vi "Autonomous Independent.vi"() -> ()   [LabVIEW 2011]
doc: "This VI is called when autonomous begins, and will automatically be terminated when autonomous ends. You can carry out timed or sensor driven robot movement independently without needing to return to the caller."
uses:
  Robot Global Data.vi
  <vilib>/addons/control/pid/pid.llb/PID (DBL).vi
  <vilib>/Rock Robotics/WPI/Solenoid/Deprecated/WPI_SolenoidSetBool.vi
  <vilib>/addons/control/pid/NI_PID_pid.lvlib
panel:
  out "Auto State":T1(ring)
  out "Right":bool
  out "Center":bool
  out "Left":bool
  out "Mast encoder":dbl
  out "Drive train encoder":dbl
  out "gyro":dbl
  in  "Steering Gain":dbl=0.6
  # "Double line at end -- the T"
  # "This picture represents the robot following the left edge\nof the line.\nIt attempts to keep an edge sensor on the line,\nand all others off. This gives it three meaningful responses,\nsteer left, steer right, and go straight.\nThis allows for the other edge sensor to be used primarily\nfor identifying the T at the end of the line."
  # "Robot"
  # "Line"
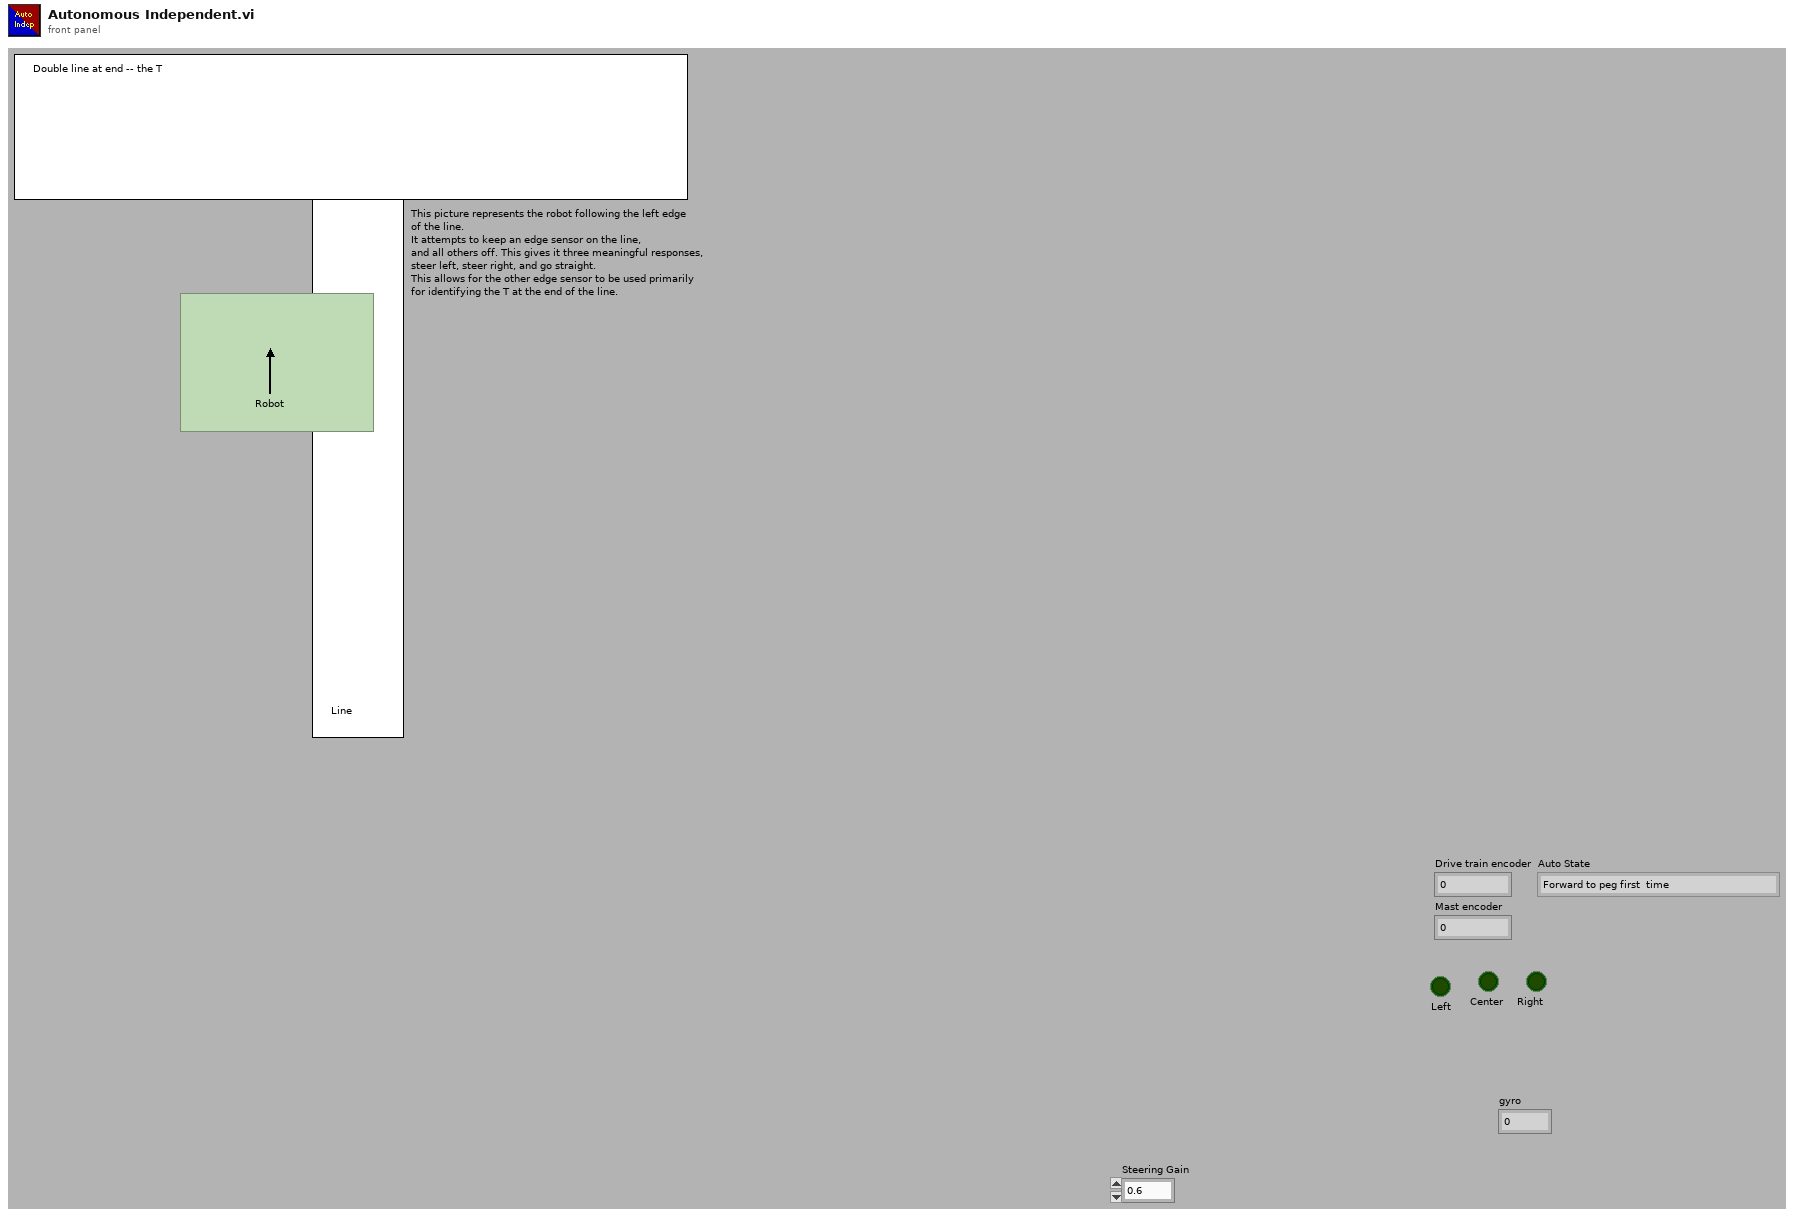
[diagram p1: front panel]
types:
  T1 = enum16{"Forward to peg first  time", "Lower Mast", "Open jaw", "Lower Mast again", "Back to second tube", "Spin to tube", "Forward to second tube", "Close jaw and forward", "Spin to zero gyro, face peg", "Forward to peg second time", "Lower mast 2", "Lower mast 3"}
  T2 = typedef "WPI_ServoDeviceRef.ctl" = cluster{"DeviceStatus":errorcluster, "Digital Module":T3, "PWM Channel":T4, "DeadBand":T5}
  T3 = typedef "FPGA_TypedefDigitalModule.ctl" = enum16{"Digital Module 1", "Digital Module 2"}
  T4 = typedef "FPGA_DIOPWMChannel.ctl" = enum8{"PWM 1", "PWM 2", "PWM 3", "PWM 4", "PWM 5", "PWM 6", "PWM 7", "PWM 8", "PWM 9", "PWM 10", "Invalid"}
  T5 = typedef "WPI_PWMDeadband.ctl" = cluster{"Name":string, "maxPositivePwm":i32, "minPositivePwm":i32, "centerPwm":i32, "maxNegativePwm":i32, "minNegativePwm":i32, "angularRange":u16}
  T6 = typedef "WPI_DigitalInputDevRef.ctl" = cluster{"DevStatus":errorcluster, "DIO Channel":T7, "Digital Module":T3}
  T7 = typedef "FPGA_DIOChannel.ctl" = enum8{"DIO 1", "DIO 2", "DIO 3", "DIO 4", "DIO 5", "DIO 6", "DIO 7", "DIO 8", "DIO 9", "DIO 10", "DIO 11", "DIO 12", "DIO 13", "DIO 14", "Invalid"}
  T8 = typedef "WPI_EncoderDevRef.ctl" = cluster{"DevStatus":errorcluster, "EncoderIndex":T9, "CounterIndex":T10, "DistancePerCount":dbl, "Decoding Type":T11}
  T9 = typedef "FPGA_EncoderIdx.ctl" = enum8{"Enc 0", "Enc 1", "Enc 2", "Enc 3", "Invalid"}
  T10 = typedef "FPGA_CounterCtrSystemIndex.ctl" = enum8{"Ctr 0", "Ctr 1", "Ctr 2", "Ctr 3", "Ctr 4", "Ctr 5", "Ctr 6", "Ctr 7", "Invalid"}
  T11 = typedef "WPI_EncoderType.ctl" = enum16{"1x", "2x", "4x"}
  T12 = typedef "WPI_RobotDriveDevRef.ctl" = cluster{"DevStatus":errorcluster, "Motors[]":T13[], "Square Inputs":bool, "Max Output":dbl}
  T13 = typedef "WPI_MotorControlDeviceRef.ctl" = cluster{"DeviceStatus":errorcluster, "Type":enum16{"PWM", "CAN"}, "PWM":cluster{"Digital Module":T3, "PWM Channel":T4, "DeadBand":T5}, "CAN":cluster{"Device Number":u8, "Control Mode":T14, "Semaphore":T15, "Max Vout":dbl}, "Invert":bool, "TransformRef":T16, "InvTransformRef":T16}
  T14 = typedef "WPI_CANJaguar_ControlMode.ctl" = enum8{"Percent VBus", "Current", "Speed", "Position", "Voltage"}
  T15 = typedef "Semaphore RefNum" = refnum<k1>
  T16 = typedef "WPI_PWMTransform_ConPane.ctl" = refnum<vi>
  T17 = typedef "WPI_GyroDevRef.ctl" = cluster{"DevStatus":errorcluster, "Analog Module":T18, "Analog Channel":T19, "Offset":dbl, "Gain (VoltsPerDegree/Second)":dbl}
  T18 = typedef "FPGA_TypedefAnalogModule.ctl" = enum16{"Analog Module 1", "Analog Module 2"}
  T19 = typedef "FPGA_AIChannel.ctl" = enum8{"AI 1", "AI 2", "AI 3", "AI 4", "AI 5", "AI 6", "AI 7", "AI 8", "Invalid"}
  T20 = typedef "WPI_SolenoidDevRef.ctl" = cluster{"DevStatus":errorcluster, "Solenoid Module":T21, "Forward Solenoid Channel":T22, "Reverse Solenoid Channel":T22}
  T21 = typedef "FPGA_TypedefSolenoidModule.ctl" = enum16{"Solenoid Module 1", "Solenoid Module 2"}
  T22 = typedef "WPI_SolenoidChannel.ctl" = enum8{"Solenoid 1", "Solenoid 2", "Solenoid 3", "Solenoid 4", "Solenoid 5", "Solenoid 6", "Solenoid 7", "Solenoid 8", "Invalid"}
  T23 = cluster{"Left":bool, "Center":bool, "Right":bool}
  T24 = cluster{"proportional gain (Kc)":dbl, "integral time (Ti, min)":dbl, "derivative time (Td, min)":dbl}
  T25 = enum16{"Forward to peg first  time", "Lower Mast", "Open jaw", "Lower Mast again", "Back to second tube", "Spin to tube", "Forward to second tube", "Close jaw and forward", "Spin to zero gyro, face peg", "Forward to peg second time", "Lower mast 2", "Lower mast 3", "Stop"}
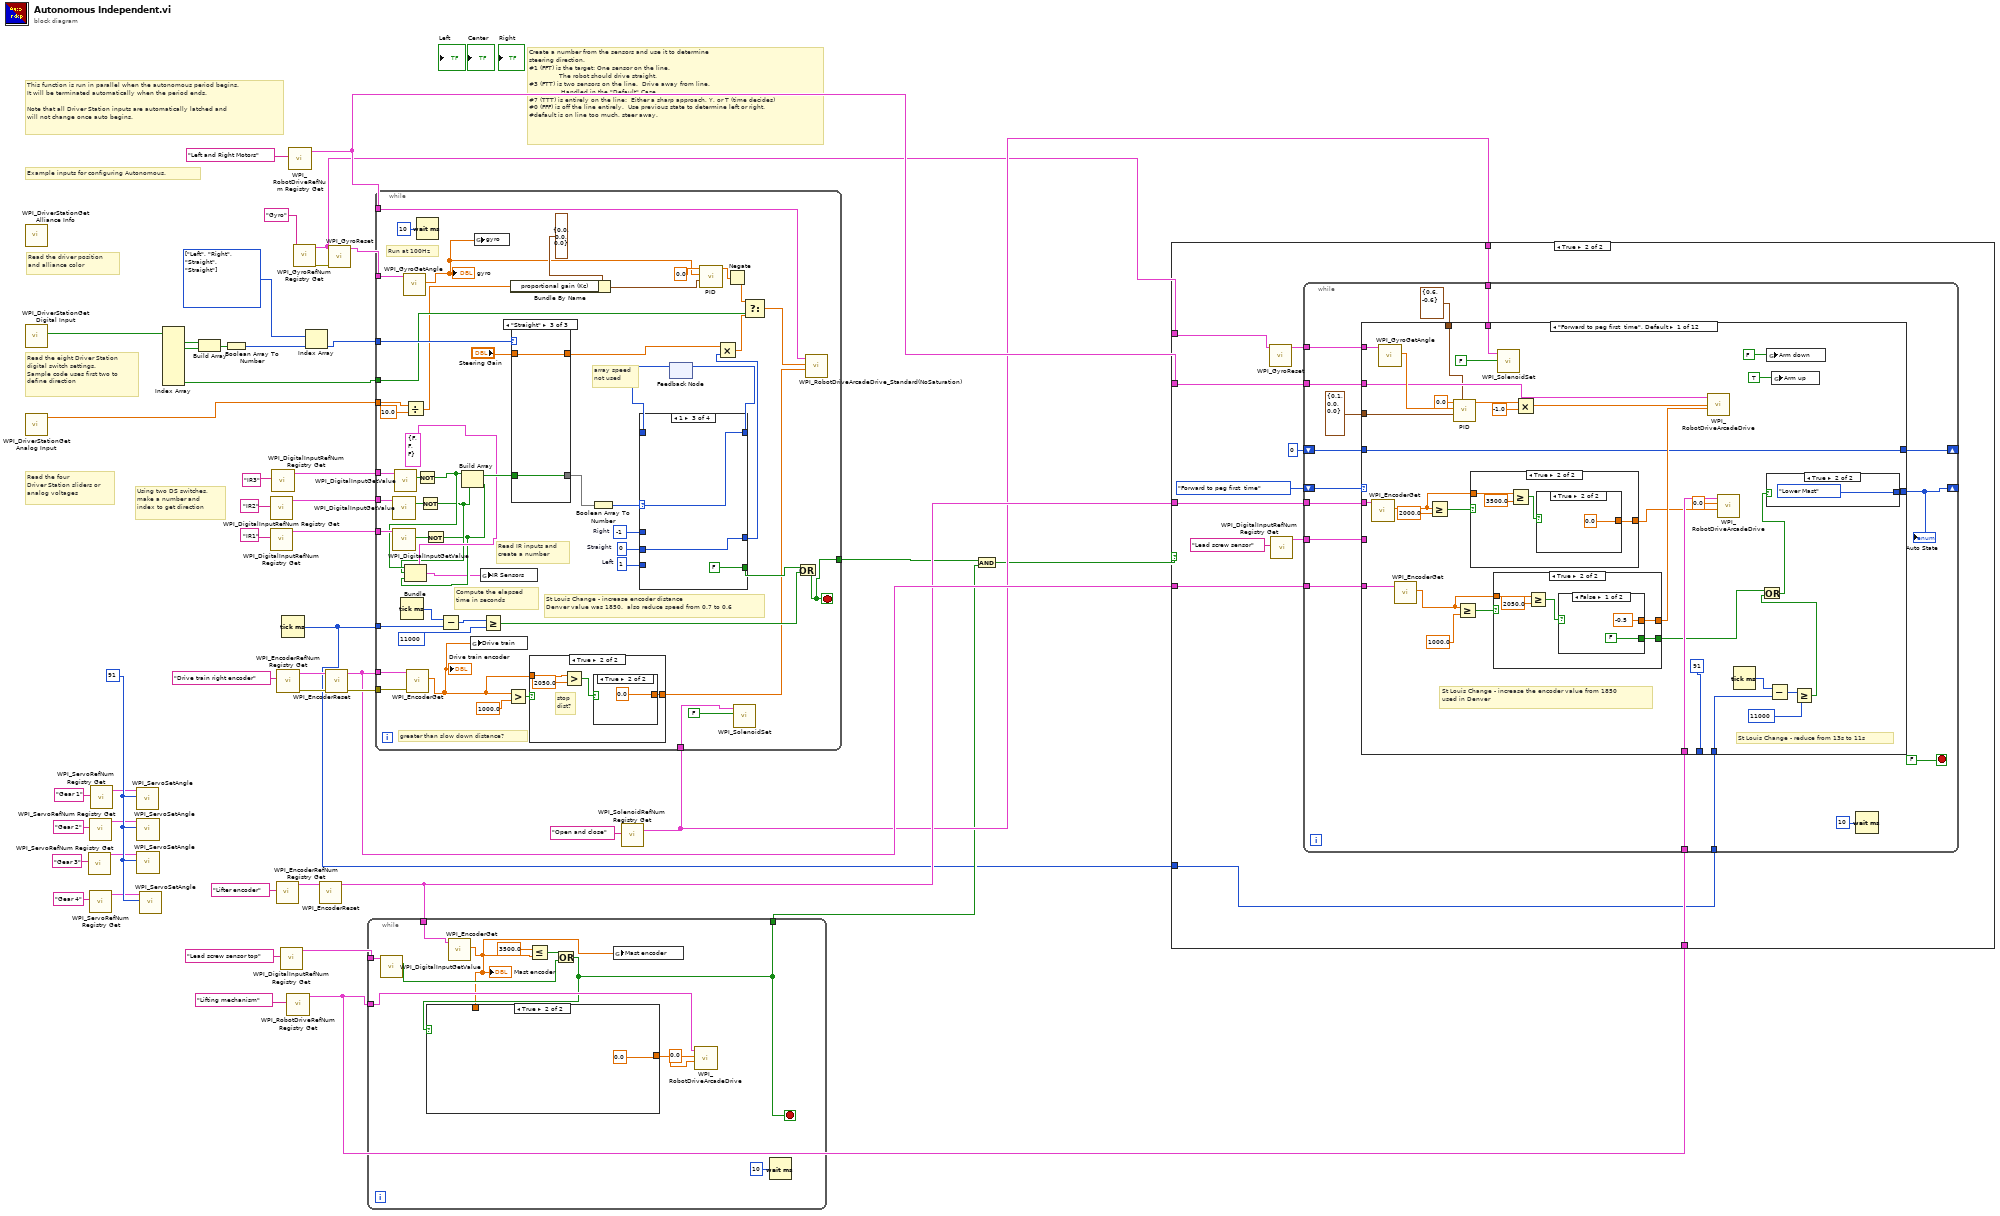
[diagram p0: block diagram]
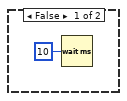
[diagram p2: hidden frame]
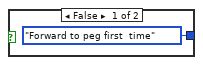
[diagram p3: hidden frame]
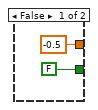
[diagram p4: hidden frame]
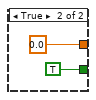
[diagram p5: hidden frame]
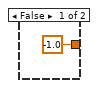
[diagram p6: hidden frame]
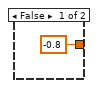
[diagram p7: hidden frame]
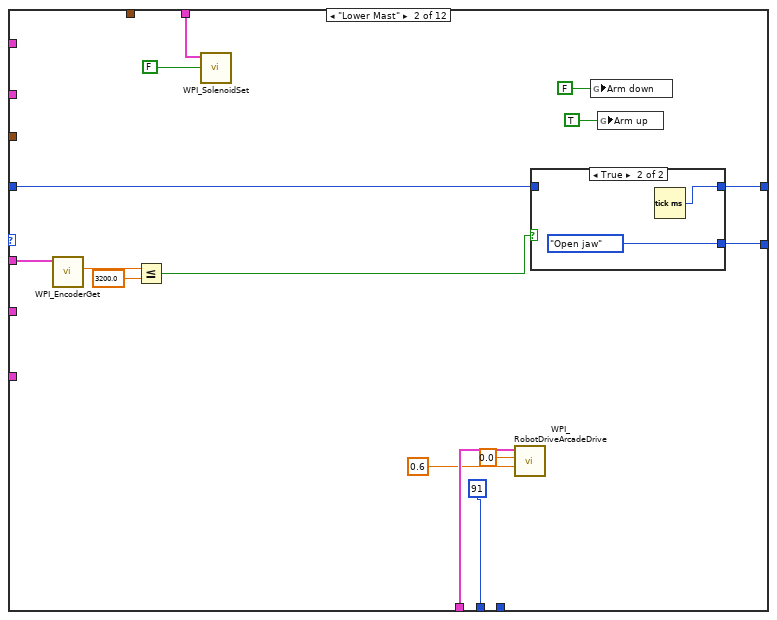
[diagram p8: hidden frame]
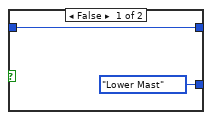
[diagram p9: hidden frame]
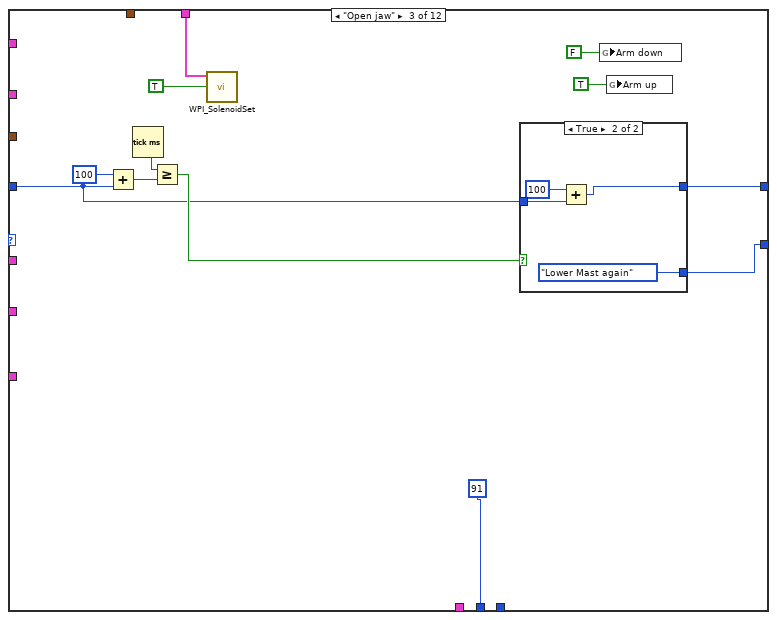
[diagram p10: hidden frame]
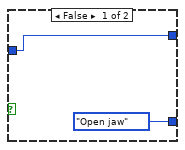
[diagram p11: hidden frame]
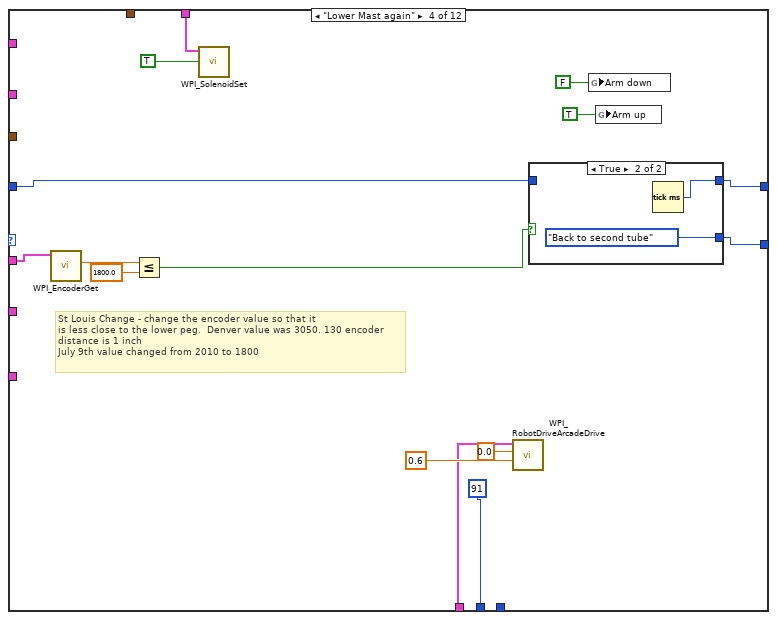
[diagram p12: hidden frame]
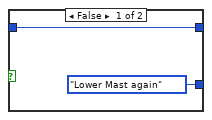
[diagram p13: hidden frame]
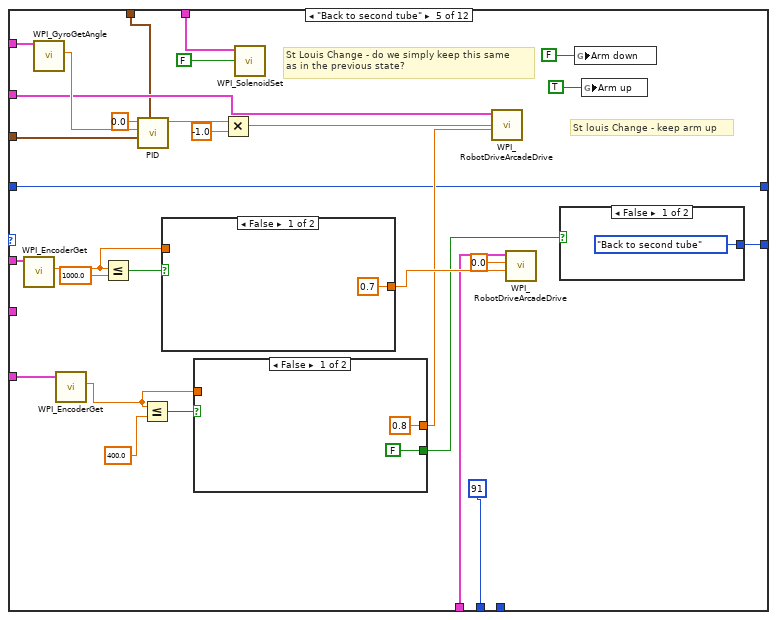
[diagram p14: hidden frame]
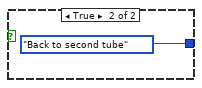
[diagram p15: hidden frame]
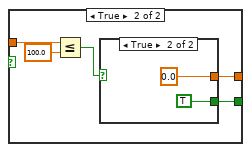
[diagram p16: hidden frame]
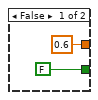
[diagram p17: hidden frame]
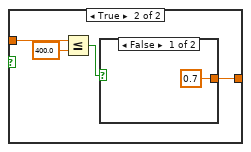
[diagram p18: hidden frame]
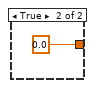
[diagram p19: hidden frame]
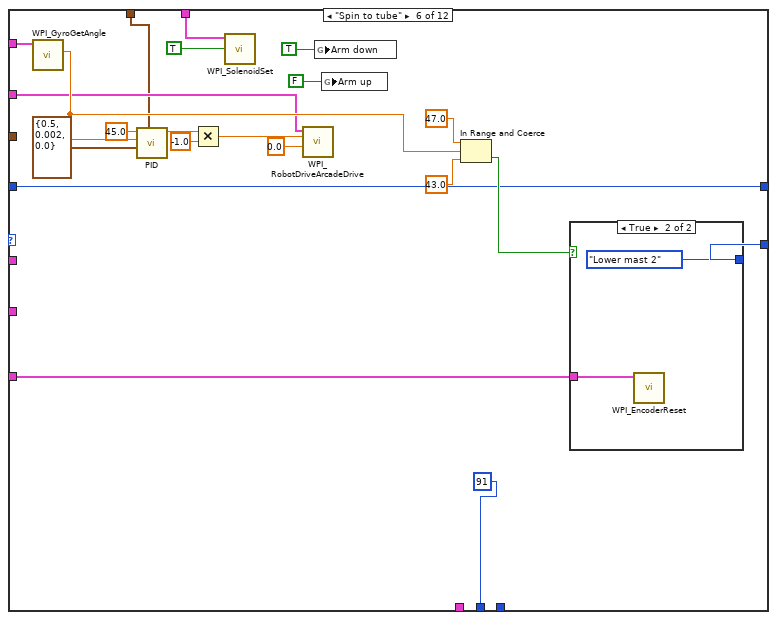
[diagram p20: hidden frame]
diagram:
  w24 = 91 ("Angle")
  w43 = enum16{"Left", "Right", "Straight"}[] [enum."Left", enum."Right", enum."Straight", enum."Straight"] items=["Left", "Right", "Straight"]
  # "Create a number from the sensors and use it to determine\nsteering direction.\n#1 (FFT) is the target: One sensor on the line.  \n               The robot should drive straight.\n#3 (FTT) is two sensors on the line.  Drive away from line.\n                Handled in the \"Default\" Case.\n#7 (TTT) is entirely on the line:  Either a sharp approach, Y, or T (time decides)\n#0 (FFF) is off the line entirely.  Use previous state to determine left or right. \n#default is on line too much, steer away."
  # "Using two DS switches,\nmake a number and\nindex to get direction"
  # "Example inputs for configuring Autonomous."
  # "Read the driver position\nand alliance color"
  # "Read the eight Driver Station\ndigital switch settings.\nSample code uses first two to\ndefine direction"
  # "Read the four\nDriver Station sliders or\nanalog voltages"
  # "This function is run in parallel when the autonomous period begins.\nIt will be terminated automatically when the period ends.\n\nNote that all Driver Station inputs are automatically latched and\nwill not change once auto begins."
  n1 = call <vilib>:"WPI_DriverStationGet Alliance Info.vi"() -> ()  [unwired: 12 out]
  n2 = call <vilib>:"WPI_DriverStationGet Digital Input.vi"() -> ("Driver Station Digital Input (1-8)"=w48:bool[])  [unwired: 11 out]
  n3 = call <vilib>:"WPI_DriverStationGet Analog Input.vi"() -> ("Analog 1 (V)"=w1:dbl)  [unwired: 11 out]
  n4 = call <vilib>:"WPI_ServoRefNum Registry Get.vi"("refnum name"="Gear 3") -> ("ServoDeviceRef"=w17:T2)  [unwired: 1 in, 9 out]
  n5 = call <vilib>:"WPI_ServoRefNum Registry Get.vi"("refnum name"="Gear 2") -> ("ServoDeviceRef"=w18:T2)  [unwired: 1 in, 9 out]
  n6 = call <vilib>:"WPI_ServoRefNum Registry Get.vi"("refnum name"="Gear 4") -> ("ServoDeviceRef"=w16:T2)  [unwired: 1 in, 9 out]
  n7 = call <vilib>:"WPI_ServoRefNum Registry Get.vi"("refnum name"="Gear 1") -> ("ServoDeviceRef"=w19:T2)  [unwired: 1 in, 9 out]
  n8 = call <vilib>:"WPI_ServoSetAngle.vi"("Angle"=w24, "ServoDeviceRef"=w19) -> ()  [unwired: 1 in, 9 out]
  n9 = call <vilib>:"WPI_ServoSetAngle.vi"("Angle"=w24, "ServoDeviceRef"=w18) -> ()  [unwired: 1 in, 9 out]
  n10 = call <vilib>:"WPI_ServoSetAngle.vi"("Angle"=w24, "ServoDeviceRef"=w17) -> ()  [unwired: 1 in, 9 out]
  n11 = call <vilib>:"WPI_ServoSetAngle.vi"("Angle"=w24, "ServoDeviceRef"=w16) -> ()  [unwired: 1 in, 9 out]
  n12 = Index Array(array=w48) -> (element #1=w46:bool, element #2=w45:bool, element #8=w4:bool)  [unwired: 8 in, 5 out]
  n13 = Build Array(w46, w45) -> (w44:bool[])
  n14 = Boolean Array To Number(Boolean array=w44) -> (number=w42:u32)
  n15 = call <vilib>:"WPI_DigitalInputRefNum Registry Get.vi"("refnum name"="IR2") -> ("DigitalInputDevRef"=w29:T6)  [unwired: 1 in, 9 out]
  n16 = call <vilib>:"WPI_DigitalInputRefNum Registry Get.vi"("refnum name"="IR1") -> ("DigitalInputDevRef"=w28:T6)  [unwired: 1 in, 9 out]
  n17 = call <vilib>:"WPI_DigitalInputRefNum Registry Get.vi"("refnum name"="IR3") -> ("DigitalInputDevRef"=w30:T6)  [unwired: 1 in, 9 out]
  n18 = call <vilib>:"WPI_EncoderRefNum Registry Get.vi"("refnum name"="Lifter encoder") -> ("EncoderDevRef"=w25:T8)  [unwired: 1 in, 9 out]
  n19 = call <vilib>:"WPI_EncoderRefNum Registry Get.vi"("refnum name"="Drive train right encoder") -> ("error out"=w32:errorcluster, "EncoderDevRef"=w31:T8)  [unwired: 1 in, 8 out]
  n20 = call <vilib>:"WPI_DigitalInputRefNum Registry Get.vi"("refnum name"="Lead screw sensor top") -> ("DigitalInputDevRef"=w26:T6)  [unwired: 1 in, 9 out]
  n21 = Tick Count (ms)() -> (millisecond timer value=w8:u32)
  n22 = call <vilib>:"WPI_RobotDriveRefNum Registry Get.vi"("refnum name"="Lifting mechanism") -> ("RobotDriveDevRef"=w14:T12)  [unwired: 1 in, 9 out]
  n23 = call <vilib>:"WPI_RobotDriveRefNum Registry Get.vi"("refnum name"="Left and Right Motors") -> ("RobotDriveDevRef"=w15:T12)  [unwired: 1 in, 9 out]
  n24 = call <vilib>:"WPI_GyroRefNum Registry Get.vi"("refnum name"="Gyro") -> ("error out"=w7:errorcluster, "GyroDevRef"=w3:T17)  [unwired: 1 in, 8 out]
  n25 = Index Array(array=w43, index=w42) -> (element=w37:enum16{"Left", "Right", "Straight"})
  n26 = call <vilib>:"WPI_EncoderReset.vi"("EncoderDevRef"=w25) -> ("EncoderDevRef"=w12:T8)  [unwired: 1 in, 9 out]
  n27 = call <vilib>:"WPI_EncoderReset.vi"("error in (no error)"=w32, "EncoderDevRef"=w31) -> ("error out"=w27:errorcluster, "EncoderDevRef"=w13:T8)  [unwired: 8 out]
  n28 = call <vilib>:"WPI_GyroReset.vi"("error in (no error)"=w7, "GyroDevRef"=w3) -> ("GyroDevRef"=w5:T17)  [unwired: 9 out]
  n29 = while {
    tunnel: w14 -> [w57]
    tunnel: w26 -> [w59]
    tunnel: [w51] -> w10
    tunnel: w12 -> [w56]
    stop <- w51 stop-if-true
    n30 = call <vilib>:"WPI_DigitalInputGetValue.vi"("DigitalInputDevRef"=w59) -> ("Value"=w52:bool)  [unwired: 1 in, 9 out]
    n31 = call <vilib>:"WPI_EncoderGet.vi"("EncoderDevRef"=w56) -> ("Distance"=w50:dbl)  [unwired: 1 in, 9 out]
    "Mast encoder" <- w50
    n32 = Less Or Equal?(x=3500.0, y=w50) -> (x <= y?=w53:bool)
    n33 = Or(x=w53, y=w52) -> (x .or. y?=w51:bool)
    n34 = case shown="True" w51 {
      tunnel: [w63 0.0 ("Y axis value")] -> w55
      tunnel: w50 -> [w60 _]
      frame False {
        # "slow down if encoder is 2700"
        n35 = Greater Or Equal?(x=w60, y=2700.0) -> (x >= y?=w62:bool)
        n36 = case shown="True" w62 {
          tunnel: [-1.0 ("Y axis value") -0.6 ("Y axis value")] -> w63
          frame False {
          }
          frame True {
          }
        }
      }
      frame True {
      }
    }
    n37 = global write "Robot Global Data.vi" "Mast encoder"(w50) -> ()
    n38 = call-poly <vilib>:"WPI_RobotDriveArcadeDrive.vi"("Y axis value"=w55, "X axis value"=0.0, "RobotDriveDevRef"=w57) -> ()  [unwired: 1 in, 8 out]
    n39 = Wait (ms)(milliseconds to wait=u32 10) -> ()  [unwired: 1 out]
  }
  n40 = call <vilib>:"WPI_SolenoidRefNum Registry Get.vi"("refnum name"="Open and close") -> ("SolenoidDevRef"=w11:T20)  [unwired: 1 in, 9 out]
  n41 = while {
    tunnel: w15 -> [w99]
    tunnel: w30 -> [w119]
    tunnel: w29 -> [w118]
    tunnel: w28 -> [w117]
    tunnel: w8 -> [w78]
    tunnel: w37 -> [w103]
    tunnel: w13 -> [w98]
    tunnel: w27 -> [w97]
    tunnel: w11 -> [w93]
    tunnel: w5 -> [w92]
    tunnel: w4 -> [w86]
    tunnel: [w75] -> w2
    tunnel: w1 -> [w72]
    stop <- w75 stop-if-true
    w111 = 0  # Straight
    w110 = 1  # Left
    w112 = -1  # Right
    # "St Louis Change - increase encoder distance \nDenver value was 1850.  also reduce speed from 0.7 to 0.6"
    # "array speed\nnot used"
    # "greater than slow down distance?"
    # "Run at 100Hz"
    # "Read IR inputs and\ncreate a number"
    # "Compute the elapsed\ntime in seconds"
    n42 = call <vilib>:"WPI_DigitalInputGetValue.vi"("DigitalInputDevRef"=w118) -> ("Value"=w101:bool)  [unwired: 1 in, 9 out]
    n43 = call <vilib>:"WPI_DigitalInputGetValue.vi"("DigitalInputDevRef"=w117) -> ("Value"=w100:bool)  [unwired: 1 in, 9 out]
    n44 = call <vilib>:"WPI_DigitalInputGetValue.vi"("DigitalInputDevRef"=w119) -> ("Value"=w102:bool)  [unwired: 1 in, 9 out]
    n45 = Tick Count (ms)() -> (millisecond timer value=w109:u32)
    n46 = call <vilib>:"WPI_GyroGetAngle.vi"("GyroDevRef"=w92) -> ("Angle"=w85:dbl)  [unwired: 1 in, 9 out]
    "gyro" <- w85
    n47 = Divide(x=w72, y=10.0) -> (x/y=w71:dbl)
    n48 = call <vilib>:"WPI_EncoderGet.vi"("error in (no error)"=w97, "EncoderDevRef"=w98) -> ("Distance"=w69:dbl)  [unwired: 9 out]
    "Drive train encoder" <- w69
    n49 = Not(x=w102) -> (.not. x?=w83:bool)
    n50 = Wait (ms)(milliseconds to wait=u32 10) -> ()  [unwired: 1 out]
    n51 = Not(x=w101) -> (.not. x?=w82:bool)
    n52 = Not(x=w100) -> (.not. x?=w81:bool)
    n53 = Bundle(cluster=T23 {"Left"=FALSE, "Center"=FALSE, "Right"=FALSE} ("IR Sensors"), "Left"=w83, "Center"=w82, "Right"=w81) -> (w80:T23)
    n54 = Subtract(x=w109, y=w78) -> (x-y=w77:u32)
    n55 = Build Array(w83, w82, w81) -> (w108:bool[])
    n56 = global write "Robot Global Data.vi" "Drive train"(w69) -> ()
    n57 = global write "Robot Global Data.vi" "gyro"(w85) -> ()
    n58 = global write "Robot Global Data.vi" "IR Sensors"(w80) -> ()
    n59 = Greater Or Equal?(x=w77, y=u32 11000 ("milliseconds to wait")) -> (x >= y?=w76:bool)
    n60 = Greater?(x=w69, y=1000.0) -> (0:w95:bool)
    n61 = Bundle By Name(cluster=T24 {"proportional gain (Kc)"=0.0, "integral time (Ti, min)"=0.0, "derivative time (Td, min)"=0.0} ("PID gains"), "proportional gain (Kc)"=w71) -> (w89:T24)
    n62 = case shown="\"Straight\"" w103 {
      tunnel: w108 -> [w127 w130 w133]
      tunnel: [w127 w129 w133] -> w107
      tunnel: "Steering Gain" -> [w128 w132 w134]
      tunnel: [w128 w131 w134] -> w104
      frame "Left", Default {
      }
      frame "Right" {
        n63 = Negate(x=w132) -> (-x=w131:dbl)
        n64 = Reverse 1D Array(array=w130) -> (reversed array=w129:bool[])
      }
      frame "Straight" {
      }
    }
    n65 = case shown="True" w95 {
      tunnel: [-0.7 ("Y axis value") w123] -> w74
      tunnel: w69 -> [_ w121]
      frame False {
      }
      frame True {
        # "stop\ndist?"
        n66 = Greater?(x=w121, y=2050.0) -> (0:w122:bool)
        n67 = case shown="True" w122 {
          tunnel: [-0.5 ("Y axis value") 0.0 ("Y axis value")] -> w123
          frame False {
          }
          frame True {
          }
        }
      }
    }
    n68 = Boolean Array To Number(Boolean array=w107) -> (number=w116:u32)
    n69 = feedback #1() -> (w115:u32)  [unwired: 1 out]
    n70 = case shown="1" w116 {
      selector: w116 -> [w136 _ w147 w150]
      tunnel: w112 -> [_ w140 _ _]
      tunnel: w111 -> [_ _ w148 w151]
      tunnel: w110 -> [w137 w141 _ _]
      tunnel: [w137 w139 w148 w151] -> w106
      tunnel: w115 -> [_ w142 _ _]
      tunnel: [w136 w142 w147 w150] -> w114
      tunnel: [FALSE FALSE FALSE TRUE] -> w79
      frame Default {
      }
      frame 0 {
        # "#1-exited on right\n#7-inside Y\n#0 initial condition"
        n71 = case shown="0, 1" w142 {
          tunnel: w141 -> [w143 _ w145]
          tunnel: w140 -> [_ w144 _]
          tunnel: [w143 w144 w145] -> w139
          frame Default {
          }
          frame 0, 1 {
          }
          frame 7 {
          }
        }
      }
      frame 1 {
      }
      frame 7 {
      }
    }
    n72 = feedback-in #1(w114) -> ()
    n73 = call-poly <vilib>:"PID.vi"("PID gains"=w89, "process variable"=w85, "setpoint"=0.0) -> ("output"=w68:dbl)  [unwired: 3 in, 5 out]
    n74 = Multiply(x=w104, y=w106) -> (x*y=w88:dbl)
    n75 = Negate(x=w68) -> (-x=w67:dbl)
    n76 = call-poly <vilib>:"WPI_SolenoidSet.vi"("Value"=FALSE, "SolenoidDevRef"=w93) -> ()  [unwired: 1 in, 9 out]
    n77 = Select(t=w67, s=w86, f=w88) -> (s? t:f=w87:dbl)
    n78 = Or(x=w79, y=w76) -> (x .or. y?=w75:bool)
    n79 = call <vilib>:"WPI_RobotDriveArcadeDrive_Standard(NoSaturation).vi"("Y axis value"=w74, "X axis value"=w87, "RobotDriveDevRef"=w99) -> ()  [unwired: 1 in, 8 out]
  }
  n80 = And(x=w2, y=w10) -> (x .and. y?=w9:bool)
  n81 = case shown="True" w9 {
    tunnel: w15 -> [_ w159]
    tunnel: w14 -> [_ w158]
    tunnel: w13 -> [_ w157]
    tunnel: w12 -> [_ w156]
    tunnel: w11 -> [_ w155]
    tunnel: w8 -> [_ w154]
    tunnel: w3 -> [_ w153]
    frame False {
      n82 = Wait (ms)(milliseconds to wait=u32 10) -> ()  [unwired: 1 out]
    }
    frame True {
      n83 = call <vilib>:"WPI_GyroReset.vi"("GyroDevRef"=w153) -> ("GyroDevRef"=w163:T17)  [unwired: 10 out]
      n84 = call <vilib>:"WPI_DigitalInputRefNum Registry Get.vi"("refnum name"="Lead screw sensor") -> ("DigitalInputDevRef"=w160:T6)  [unwired: 1 in, 9 out]
      n85 = while {
        shift-right: [w172] -> _
        shift-left: T25."Forward to peg first  time" -> [w179]
        tunnel: w163 -> [w178]
        tunnel: w159 -> [w176]
        tunnel: w157 -> [w175]
        tunnel: w156 -> [w174]
        tunnel: w158 -> [w173]
        shift-right: [w170] -> _
        shift-left: u32 0 ("millisecond timer value") -> [w171]
        tunnel: w155 -> [w169]
        tunnel: w160 -> [w168]
        tunnel: w154 -> [w166]
        stop <- FALSE stop-if-true
        n86 = case shown="\"Forward to peg first  time\", Default" w179 {
          tunnel: w178 -> [w215 _ _ _ w303 w356 w383 w411 w435 w462 _ _]
          tunnel: T24 {"proportional gain (Kc)"=0.1, "integral time (Ti, min)"=0.0, "derivative time (Td, min)"=0.0} ("PID gains") -> [w212 _ _ _ w302 _ w384 w410 _ w460 _ _]
          tunnel: w176 -> [w211 _ _ _ w304 w344 w382 w412 w434 w461 _ _]
          tunnel: w175 -> [w210 _ _ _ w299 w343 w377 w407 w430 w458 _ _]
          tunnel: w174 -> [w209 w250 _ w278 w295 _ _ _ _ w459 w505 w524]
          tunnel: w173 -> [w202 w245 _ w275 w300 _ w366 _ _ w456 w508 w521]
          tunnel: [w199 w246 w263 w277 w297 w347 w374 w403 w431 w455 w506 T1."Lower mast 3"] -> w172
          tunnel: w171 -> [w196 w239 w261 w279 w301 w345 w375 w405 w433 w457 w509 _]
          tunnel: [w196 w240 w260 w276 w301 w345 w375 w405 w433 w457 w507 u32 0 ("millisecond timer value")] -> w170
          tunnel: w169 -> [w194 w237 w259 w274 w296 w353 w385 w413 w436 w463 w501 w528]
          tunnel: w168 -> [_ _ _ _ _ _ w367 _ _ _ _ _]
          tunnel: cluster{"output high":dbl, "output low":dbl} {"output high"=0.6, "output low"=-0.6} ("output range") -> [w190 _ _ _ w294 w342 w372 w402 w429 w454 _ _]
          tunnel: [91 ("Angle") 91 ("Angle") 91 ("Angle") 91 ("Angle") 91 ("Angle") 91 ("Angle") 91 ("Angle") 91 ("Angle") 91 ("Angle") 91 ("Angle") 91 ("Angle") 91 ("Angle")] -> _
          tunnel: w166 -> [w186 _ _ _ _ _ _ _ _ _ _ _]
          frame "Forward to peg first  time", Default {
            # "St Louis Change - reduce from 13s to 11s"
            # "St Louis Change - increase the encoder value from 1850\nused in Denver"
            n87 = call <vilib>:"WPI_EncoderGet.vi"("EncoderDevRef"=w209) -> ("Distance"=w200:dbl)  [unwired: 1 in, 9 out]
            n88 = call <vilib>:"WPI_GyroGetAngle.vi"("GyroDevRef"=w215) -> ("Angle"=w214:dbl)  [unwired: 1 in, 9 out]
            n89 = call <vilib>:"WPI_EncoderGet.vi"("EncoderDevRef"=w210) -> ("Distance"=w188:dbl)  [unwired: 1 in, 9 out]
            n90 = Greater Or Equal?(x=w200, y=2000.0) -> (x >= y?=w207:bool)
            n91 = call-poly <vilib>:"PID.vi"("output range"=w190, "PID gains"=w212, "process variable"=w214, "setpoint"=0.0) -> ("output"=w193:dbl)  [unwired: 2 in, 5 out]
            n92 = Greater Or Equal?(x=w188, y=1000.0) -> (x >= y?=w206:bool)
            n93 = case shown="True" w207 {
              tunnel: [-1.0 ("Y axis value") w233] -> w201
              tunnel: w200 -> [_ w232]
              frame False {
              }
              frame True {
                n94 = Greater Or Equal?(x=w232, y=3500.0) -> (x >= y?=w230:bool)
                n95 = case shown="True" w230 {
                  tunnel: [-0.8 ("Y axis value") 0.0 ("Y axis value")] -> w233
                  frame False {
                  }
                  frame True {
                  }
                }
              }
            }
            n96 = case shown="True" w206 {
              tunnel: [-0.5 ("Y axis value") w224] -> w204
              tunnel: w188 -> [_ w222]
              tunnel: [FALSE w220] -> w185
              frame False {
              }
              frame True {
                n97 = Greater Or Equal?(x=w222, y=2050.0) -> (x >= y?=w223:bool)
                n98 = case shown="False" w223 {
                  tunnel: [-0.5 ("Y axis value") 0.0 ("Y axis value")] -> w224
                  tunnel: [FALSE TRUE] -> w220
                  frame False {
                  }
                  frame True {
                  }
                }
              }
            }
            n99 = call-poly <vilib>:"WPI_SolenoidSet.vi"("Value"=FALSE, "SolenoidDevRef"=w194) -> ()  [unwired: 1 in, 9 out]
            n100 = Multiply(x=w193, y=-1.0) -> (x*y=w191:dbl)
            n101 = call-poly <vilib>:"WPI_RobotDriveArcadeDrive.vi"("Y axis value"=w204, "X axis value"=w191, "RobotDriveDevRef"=w211) -> ()  [unwired: 1 in, 8 out]
            n102 = call-poly <vilib>:"WPI_RobotDriveArcadeDrive.vi"("Y axis value"=w201, "X axis value"=0.0, "RobotDriveDevRef"=w202) -> ()  [unwired: 1 in, 8 out]
            n103 = Tick Count (ms)() -> (millisecond timer value=w187:u32)
            n104 = global write "Robot Global Data.vi" "Arm down"(FALSE ("Arm down")) -> ()
            n105 = Subtract(x=w187, y=w186) -> (x-y=w184:u32)
            n106 = global write "Robot Global Data.vi" "Arm up"(TRUE ("Arm up")) -> ()
            n107 = Greater Or Equal?(x=w184, y=u32 11000) -> (x >= y?=w182:bool)
            n108 = Or(x=w185, y=w182) -> (x .or. y?=w181:bool)
            n109 = case shown="True" w181 {
              tunnel: [T1."Forward to peg first  time" T1."Lower Mast"] -> w199
              frame False {
              }
              frame True {
              }
            }
          }
          frame "Lower Mast" {
            n110 = call <vilib>:"WPI_EncoderGet.vi"("EncoderDevRef"=w250) -> ("Distance"=w249:dbl)  [unwired: 1 in, 9 out]
            n111 = Less Or Equal?(x=w249, y=3200.0) -> (x <= y?=w247:bool)
            n112 = call-poly <vilib>:"WPI_SolenoidSet.vi"("Value"=FALSE, "SolenoidDevRef"=w237) -> ()  [unwired: 1 in, 9 out]
            n113 = call-poly <vilib>:"WPI_RobotDriveArcadeDrive.vi"("Y axis value"=0.6, "X axis value"=0.0, "RobotDriveDevRef"=w245) -> ()  [unwired: 1 in, 8 out]
            n114 = case shown="True" w247 {
              tunnel: [T1."Lower Mast" T1."Open jaw"] -> w246
              tunnel: [w251 w253] -> w240
              tunnel: w239 -> [w251 _]
              frame False {
              }
              frame True {
                n115 = Tick Count (ms)() -> (millisecond timer value=w253:u32)
              }
            }
            n116 = global write "Robot Global Data.vi" "Arm down"(FALSE ("Arm down")) -> ()
            n117 = global write "Robot Global Data.vi" "Arm up"(TRUE ("Arm up")) -> ()
          }
          frame "Open jaw" {
            n118 = Add(x=u32 100, y=w261) -> (x+y=w265:u32)
            n119 = Tick Count (ms)() -> (millisecond timer value=w264:u32)
            n120 = Greater Or Equal?(x=w264, y=w265) -> (x >= y?=w262:bool)
            n121 = call-poly <vilib>:"WPI_SolenoidSet.vi"("Value"=TRUE, "SolenoidDevRef"=w259) -> ()  [unwired: 1 in, 9 out]
            n122 = case shown="True" w262 {
              tunnel: [T1."Open jaw" T1."Lower Mast again"] -> w263
              tunnel: w261 -> [w267 w271]
              tunnel: [w267 w269] -> w260
              frame False {
              }
              frame True {
                n123 = Add(x=u32 100, y=w271) -> (x+y=w269:u32)
              }
            }
            n124 = global write "Robot Global Data.vi" "Arm down"(FALSE ("Arm down")) -> ()
            n125 = global write "Robot Global Data.vi" "Arm up"(TRUE ("Arm up")) -> ()
          }
          frame "Lower Mast again" {
            # "St Louis Change - change the encoder value so that it\nis less close to the lower peg.  Denver value was 3050. 130 encoder\ndistance is 1 inch\nJuly 9th value changed from 2010 to 1800"
            n126 = call <vilib>:"WPI_EncoderGet.vi"("EncoderDevRef"=w278) -> ("Distance"=w280:dbl)  [unwired: 1 in, 9 out]
            n127 = Less Or Equal?(x=w280, y=1800.0) -> (x <= y?=w282:bool)
            n128 = call-poly <vilib>:"WPI_SolenoidSet.vi"("Value"=TRUE, "SolenoidDevRef"=w274) -> ()  [unwired: 1 in, 9 out]
            n129 = call-poly <vilib>:"WPI_RobotDriveArcadeDrive.vi"("Y axis value"=0.6, "X axis value"=0.0, "RobotDriveDevRef"=w275) -> ()  [unwired: 1 in, 8 out]
            n130 = case shown="True" w282 {
              tunnel: [T1."Lower Mast again" T1."Back to second tube"] -> w277
              tunnel: [w288 w290] -> w276
              tunnel: w279 -> [w288 _]
              frame False {
              }
              frame True {
                n131 = Tick Count (ms)() -> (millisecond timer value=w290:u32)
              }
            }
            n132 = global write "Robot Global Data.vi" "Arm down"(FALSE ("Arm down")) -> ()
            n133 = global write "Robot Global Data.vi" "Arm up"(TRUE ("Arm up")) -> ()
          }
          frame "Back to second tube" {
            # "St Louis Change - do we simply keep this same\nas in the previous state?"
            # "St louis Change - keep arm up"
            n134 = call <vilib>:"WPI_EncoderGet.vi"("EncoderDevRef"=w295) -> ("Distance"=w314:dbl)  [unwired: 1 in, 9 out]
            n135 = call <vilib>:"WPI_GyroGetAngle.vi"("GyroDevRef"=w303) -> ("Angle"=w305:dbl)  [unwired: 1 in, 9 out]
            n136 = call <vilib>:"WPI_EncoderGet.vi"("EncoderDevRef"=w299) -> ("Distance"=w292:dbl)  [unwired: 1 in, 9 out]
            n137 = Less Or Equal?(x=w314, y=1000.0) -> (x <= y?=w308:bool)
            n138 = call-poly <vilib>:"PID.vi"("output range"=w294, "PID gains"=w302, "process variable"=w305, "setpoint"=0.0) -> ("output"=w318:dbl)  [unwired: 2 in, 5 out]
            n139 = Less Or Equal?(x=w292, y=400.0) -> (x <= y?=w309:bool)
            n140 = case shown="False" w308 {
              tunnel: [0.7 ("Y axis value") w338] -> w313
              tunnel: w314 -> [_ w337]
              frame False {
              }
              frame True {
                n141 = Less Or Equal?(x=w337, y=400.0) -> (x <= y?=w335:bool)
                n142 = case shown="False" w335 {
                  tunnel: [0.7 ("Y axis value") 0.0 ("Y axis value")] -> w338
                  frame False {
                  }
                  frame True {
                  }
                }
              }
            }
            n143 = case shown="False" w309 {
              tunnel: [0.8 ("Y axis value") w329] -> w311
              tunnel: w292 -> [_ w327]
              tunnel: [FALSE w325] -> w298
              frame False {
              }
              frame True {
                n144 = Less Or Equal?(x=w327, y=100.0) -> (x <= y?=w328:bool)
                n145 = case shown="True" w328 {
                  tunnel: [0.6 ("Y axis value") 0.0 ("Y axis value")] -> w329
                  tunnel: [FALSE TRUE] -> w325
                  frame False {
                  }
                  frame True {
                  }
                }
              }
            }
            n146 = Multiply(x=w318, y=-1.0) -> (x*y=w320:dbl)
            n147 = call-poly <vilib>:"WPI_SolenoidSet.vi"("Value"=FALSE, "SolenoidDevRef"=w296) -> ()  [unwired: 1 in, 9 out]
            n148 = call-poly <vilib>:"WPI_RobotDriveArcadeDrive.vi"("Y axis value"=w311, "X axis value"=w320, "RobotDriveDevRef"=w304) -> ()  [unwired: 1 in, 8 out]
            n149 = call-poly <vilib>:"WPI_RobotDriveArcadeDrive.vi"("Y axis value"=w313, "X axis value"=0.0, "RobotDriveDevRef"=w300) -> ()  [unwired: 1 in, 8 out]
            n150 = case shown="False" w298 {
              tunnel: [T1."Back to second tube" T1."Back to second tube"] -> w297
              frame False {
              }
              frame True {
              }
            }
            n151 = global write "Robot Global Data.vi" "Arm down"(FALSE ("Arm down")) -> ()
            n152 = global write "Robot Global Data.vi" "Arm up"(TRUE ("Arm up")) -> ()
          }
          frame "Spin to tube" {
            n153 = call <vilib>:"WPI_GyroGetAngle.vi"("GyroDevRef"=w356) -> ("Angle"=w348:dbl)  [unwired: 1 in, 9 out]
            n154 = call-poly <vilib>:"PID.vi"("output range"=w342, "PID gains"=T24 {"proportional gain (Kc)"=0.5, "integral time (Ti, min)"=0.002, "derivative time (Td, min)"=0.0}, "process variable"=w348, "setpoint"=45.0) -> ("output"=w360:dbl)  [unwired: 2 in, 5 out]
            n155 = Multiply(x=w360, y=-1.0) -> (x*y=w358:dbl)
            n156 = call-poly <vilib>:"WPI_SolenoidSet.vi"("Value"=TRUE, "SolenoidDevRef"=w353) -> ()  [unwired: 1 in, 9 out]
            n157 = call-poly <vilib>:"WPI_RobotDriveArcadeDrive.vi"("Y axis value"=0.0, "X axis value"=w358, "RobotDriveDevRef"=w344) -> ()  [unwired: 1 in, 8 out]
            n158 = global write "Robot Global Data.vi" "Arm down"(TRUE ("Arm down")) -> ()
            n159 = global write "Robot Global Data.vi" "Arm up"(FALSE ("Arm up")) -> ()
            n160 = In Range and Coerce(upper limit=47.0, x=w348, lower limit=43.0) -> (In Range?=w346:bool)  [unwired: 1 out]
            n161 = case shown="True" w346 {
              tunnel: [T1."Spin to tube" T1."Lower mast 2"] -> w347
              tunnel: w343 -> [_ w363]
              frame False {
              }
              frame True {
                n162 = call <vilib>:"WPI_EncoderReset.vi"("EncoderDevRef"=w363) -> ()  [unwired: 1 in, 10 out]
              }
            }
          }
          frame "Forward to second tube" {
            n163 = call <vilib>:"WPI_GyroGetAngle.vi"("GyroDevRef"=w383) -> ("Angle"=w386:dbl)  [unwired: 1 in, 9 out]
            n164 = call <vilib>:"WPI_EncoderGet.vi"("EncoderDevRef"=w377) -> ("Distance"=w365:dbl)  [unwired: 1 in, 9 out]
            n165 = call-poly <vilib>:"PID.vi"("output range"=w372, "PID gains"=w384, "process variable"=w386, "setpoint"=45.0) -> ("output"=w389:dbl)  [unwired: 2 in, 5 out]
            n166 = Greater Or Equal?(x=w365, y=200.0) -> (x >= y?=w378:bool)
            n167 = call <vilib>:"WPI_DigitalInputGetValue.vi"("DigitalInputDevRef"=w367) -> ("Value"=w368:bool)  [unwired: 1 in, 9 out]
            n168 = call-poly <vilib>:"WPI_SolenoidSet.vi"("Value"=TRUE, "SolenoidDevRef"=w385) -> ()  [unwired: 1 in, 9 out]
            n169 = case shown="False" w378 {
              tunnel: [-0.7 ("Y axis value") 0.0 ("Y axis value")] -> w376
              tunnel: [FALSE TRUE] -> w373
              frame False {
              }
              frame True {
              }
            }
            n170 = Multiply(x=w389, y=-1.0) -> (x*y=w391:dbl)
            n171 = case shown="True" w368 {
              tunnel: [0.6 ("Y axis value") 0.0 ("Y axis value")] -> w370
              frame False {
              }
              frame True {
              }
            }
            n172 = global write "Robot Global Data.vi" "Arm down"(TRUE ("Arm down")) -> ()
            n173 = global write "Robot Global Data.vi" "Arm up"(FALSE ("Arm up")) -> ()
            n174 = call-poly <vilib>:"WPI_RobotDriveArcadeDrive.vi"("Y axis value"=w370, "X axis value"=0.0, "RobotDriveDevRef"=w366) -> ()  [unwired: 1 in, 8 out]
            n175 = call-poly <vilib>:"WPI_RobotDriveArcadeDrive.vi"("Y axis value"=w376, "X axis value"=w391, "RobotDriveDevRef"=w382) -> ()  [unwired: 1 in, 8 out]
            n176 = case shown="True" w373 {
              tunnel: [T1."Forward to second tube" T1."Close jaw and forward"] -> w374
              frame False {
              }
              frame True {
              }
            }
          }
          frame "Close jaw and forward" {
            n177 = call <vilib>:"WPI_GyroGetAngle.vi"("GyroDevRef"=w411) -> ("Angle"=w419:dbl)  [unwired: 1 in, 9 out]
            n178 = call <vilib>:"WPI_EncoderGet.vi"("EncoderDevRef"=w407) -> ("Distance"=w400:dbl)  [unwired: 1 in, 9 out]
            n179 = Greater Or Equal?(x=w400, y=250.0) -> (x >= y?=w409:bool)
            n180 = call-poly <vilib>:"PID.vi"("output range"=w402, "PID gains"=w410, "process variable"=w419, "setpoint"=45.0) -> ("output"=w416:dbl)  [unwired: 2 in, 5 out]
            n181 = case shown="True" w409 {
              tunnel: [-0.7 ("Y axis value") 0.0 ("Y axis value")] -> w406
              tunnel: [FALSE TRUE] -> w404
              frame False {
              }
              frame True {
              }
            }
            n182 = call-poly <vilib>:"WPI_SolenoidSet.vi"("Value"=FALSE, "SolenoidDevRef"=w413) -> ()  [unwired: 1 in, 9 out]
            n183 = Multiply(x=w416, y=-1.0) -> (x*y=w414:dbl)
            n184 = global write "Robot Global Data.vi" "Arm down"(TRUE ("Arm down")) -> ()
            n185 = global write "Robot Global Data.vi" "Arm up"(FALSE ("Arm up")) -> ()
            n186 = call-poly <vilib>:"WPI_RobotDriveArcadeDrive.vi"("Y axis value"=w406, "X axis value"=w414, "RobotDriveDevRef"=w412) -> ()  [unwired: 1 in, 8 out]
            n187 = case shown="True" w404 {
              tunnel: [T1."Close jaw and forward" T1."Spin to zero gyro, face peg"] -> w403
              frame False {
              }
              frame True {
              }
            }
          }
          frame "Spin to zero gyro, face peg" {
            n188 = call <vilib>:"WPI_GyroGetAngle.vi"("GyroDevRef"=w435) -> ("Angle"=w448:dbl)  [unwired: 1 in, 9 out]
            n189 = call-poly <vilib>:"PID.vi"("output range"=w429, "PID gains"=T24 {"proportional gain (Kc)"=0.5, "integral time (Ti, min)"=0.002, "derivative time (Td, min)"=0.0}, "process variable"=w448, "setpoint"=0.0) -> ("output"=w438:dbl)  [unwired: 2 in, 5 out]
            n190 = Multiply(x=w438, y=-1.0) -> (x*y=w440:dbl)
            n191 = call-poly <vilib>:"WPI_SolenoidSet.vi"("Value"=FALSE, "SolenoidDevRef"=w436) -> ()  [unwired: 1 in, 9 out]
            n192 = call-poly <vilib>:"WPI_RobotDriveArcadeDrive.vi"("Y axis value"=0.0, "X axis value"=w440, "RobotDriveDevRef"=w434) -> ()  [unwired: 1 in, 8 out]
            n193 = global write "Robot Global Data.vi" "Arm down"(FALSE ("Arm down")) -> ()
            n194 = global write "Robot Global Data.vi" "Arm up"(TRUE ("Arm up")) -> ()
            n195 = In Range and Coerce(upper limit=2.0, x=w448, lower limit=-2.0) -> (In Range?=w432:bool)  [unwired: 1 out]
            n196 = case shown="True" w432 {
              tunnel: [T1."Spin to zero gyro, face peg" T1."Forward to peg second time"] -> w431
              tunnel: w430 -> [_ w450]
              frame False {
              }
              frame True {
                n197 = call <vilib>:"WPI_EncoderReset.vi"("EncoderDevRef"=w450) -> ()  [unwired: 1 in, 10 out]
              }
            }
          }
          frame "Forward to peg second time" {
            n198 = call <vilib>:"WPI_EncoderGet.vi"("EncoderDevRef"=w459) -> ("Distance"=w473:dbl)  [unwired: 1 in, 9 out]
            n199 = call <vilib>:"WPI_GyroGetAngle.vi"("GyroDevRef"=w462) -> ("Angle"=w464:dbl)  [unwired: 1 in, 9 out]
            n200 = call <vilib>:"WPI_EncoderGet.vi"("EncoderDevRef"=w458) -> ("Distance"=w452:dbl)  [unwired: 1 in, 9 out]
            n201 = Greater Or Equal?(x=w473, y=2000.0) -> (x >= y?=w467:bool)
            n202 = call-poly <vilib>:"PID.vi"("output range"=w454, "PID gains"=w460, "process variable"=w464, "setpoint"=0.0) -> ("output"=w478:dbl)  [unwired: 2 in, 5 out]
            n203 = Greater Or Equal?(x=w452, y=1000.0) -> (x >= y?=w468:bool)
            n204 = case shown="True" w467 {
              tunnel: [-1.0 ("Y axis value") w498] -> w472
              tunnel: w473 -> [_ w497]
              frame False {
              }
              frame True {
                n205 = Greater Or Equal?(x=w497, y=3100.0) -> (x >= y?=w495:bool)
                n206 = case shown="True" w495 {
                  tunnel: [-0.8 ("Y axis value") 0.0 ("Y axis value")] -> w498
                  frame False {
                  }
                  frame True {
                  }
                }
              }
            }
            n207 = case shown="True" w468 {
              tunnel: [-0.8 ("Y axis value") w489] -> w470
              tunnel: [FALSE w486] -> w474
              tunnel: w452 -> [_ w485]
              frame False {
              }
              frame True {
                n208 = Greater Or Equal?(x=w485, y=1550.0) -> (x >= y?=w488:bool)
                n209 = case shown="True" w488 {
                  tunnel: [-0.6 ("Y axis value") 0.0 ("Y axis value")] -> w489
                  tunnel: [FALSE TRUE] -> w486
                  frame False {
                  }
                  frame True {
                  }
                }
              }
            }
            n210 = call-poly <vilib>:"WPI_SolenoidSet.vi"("Value"=FALSE, "SolenoidDevRef"=w463) -> ()  [unwired: 1 in, 9 out]
            n211 = Multiply(x=w478, y=-1.0) -> (x*y=w480:dbl)
            n212 = call-poly <vilib>:"WPI_RobotDriveArcadeDrive.vi"("Y axis value"=w470, "X axis value"=w480, "RobotDriveDevRef"=w461) -> ()  [unwired: 1 in, 8 out]
            n213 = call-poly <vilib>:"WPI_RobotDriveArcadeDrive.vi"("Y axis value"=w472, "X axis value"=0.0, "RobotDriveDevRef"=w456) -> ()  [unwired: 1 in, 8 out]
            n214 = case shown="False" w474 {
              tunnel: [T1."Forward to peg second time" T1."Lower mast 2"] -> w455
              frame False {
              }
              frame True {
              }
            }
            n215 = global write "Robot Global Data.vi" "Arm down"(FALSE ("Arm down")) -> ()
            n216 = global write "Robot Global Data.vi" "Arm up"(TRUE ("Arm up")) -> ()
          }
          frame "Lower mast 2" {
            n217 = call <vilib>:"WPI_EncoderGet.vi"("EncoderDevRef"=w505) -> ("Distance"=w510:dbl)  [unwired: 1 in, 9 out]
            n218 = Less Or Equal?(x=w510, y=2900.0) -> (x <= y?=w512:bool)
            n219 = call-poly <vilib>:"WPI_SolenoidSet.vi"("Value"=FALSE, "SolenoidDevRef"=w501) -> ()  [unwired: 1 in, 9 out]
            n220 = global write "Robot Global Data.vi" "Arm down"(FALSE ("Arm down")) -> ()
            n221 = global write "Robot Global Data.vi" "Arm up"(TRUE ("Arm up")) -> ()
            n222 = call-poly <vilib>:"WPI_RobotDriveArcadeDrive.vi"("Y axis value"=0.6, "X axis value"=0.0, "RobotDriveDevRef"=w508) -> ()  [unwired: 1 in, 8 out]
            n223 = case shown="False" w512 {
              tunnel: [T1."Lower Mast" T1."Open jaw"] -> w506
              tunnel: [w516 w518] -> w507
              tunnel: w509 -> [w516 _]
              frame False {
              }
              frame True {
                n224 = Tick Count (ms)() -> (millisecond timer value=w518:u32)
              }
            }
          }
          frame "Lower mast 3" {
            n225 = call <vilib>:"WPI_EncoderGet.vi"("EncoderDevRef"=w524) -> ("Distance"=w526:dbl)  [unwired: 1 in, 9 out]
            n226 = Less Or Equal?(x=w526, y=2900.0) -> (x <= y?=w520:bool)
            n227 = case shown="True" w520 {
              tunnel: [0.6 ("Y axis value") 0.0 ("Y axis value")] -> w522
              frame False {
              }
              frame True {
              }
            }
            n228 = call-poly <vilib>:"WPI_SolenoidSet.vi"("Value"=TRUE, "SolenoidDevRef"=w528) -> ()  [unwired: 1 in, 9 out]
            n229 = call-poly <vilib>:"WPI_RobotDriveArcadeDrive.vi"("Y axis value"=w522, "X axis value"=0.0, "RobotDriveDevRef"=w521) -> ()  [unwired: 1 in, 8 out]
          }
        }
        "Auto State" <- w172
        n230 = Wait (ms)(milliseconds to wait=u32 10) -> ()  [unwired: 1 out]
      }
    }
  }
